vi "INI File Path.vi"() -> (1 "ini File Path":path)   [LabVIEW 2014, in "Conventions.lvlib"]
uses:
  Conventions.lvlib
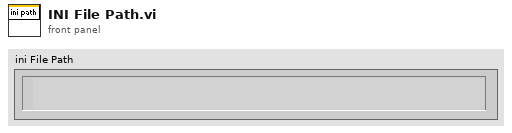
[diagram p1: front panel]
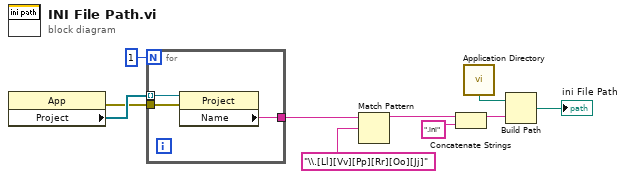
[diagram p0: block diagram]
diagram:
  n1 = property class="App"() -> (error out=w6:errorcluster, "Project"=w7:refnum<vi>[])  [unwired: 2 in, 1 out]
  n2 = for {
    N: 1 -> [_]
    tunnel: w7 -> [w13] mode=indexing
    tunnel: w6 -> [w12]
    tunnel: [w11] -> w3
    n3 = property class="Project"(reference=w13, error in=w12) -> ("Name"=w11:string)  [unwired: 2 out]
  }
  n4 = Match Pattern(string=w3, regular expression="\\.[Ll][Vv][Pp][Rr][Oo][Jj]") -> (before substring=w1:string)  [unwired: 1 in, 3 out]
  n5 = Concatenate Strings(w1, ".ini" ("string")) -> (w9:string)
  n6 = call <vilib>:"Application Directory.vi"() -> ("Application Directory"=w4:path)
  n7 = Build Path(base path=w4, name or relative path=w9) -> (appended path=→"ini File Path":path)
